vi "Animal Data Top Stack.vi"(2 "State Stack (in)":T1[](array[typedef])) -> (0 "State Stack (out)":T1[](array[typedef]), 1 "State":T1)   [LabVIEW 2016]
uses:
  Animal Data Processor state.ctl
panel:
  # "Top Stack\nVER 1.0 AAM 10th April 2002\n\nThis VI removes the top element of the state stack \nand returns the remaining elements in the stack"
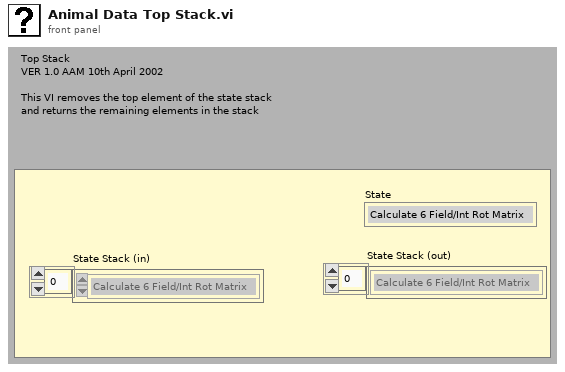
[diagram p1: front panel]
types:
  T1 = typedef "Animal Data Processor state.ctl" = enum16{"Calculate 6 Field/Int Rot Matrix", "Panel Monitoring", "Initialize", "Read 6 Field/Int Calibration File", "Read 6 Field/Int Data File", "Sort 6 Field/Int Channels", "Export Channels", "Stop", "Quit"}
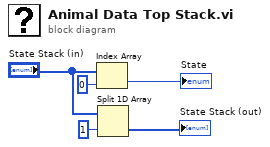
[diagram p0: block diagram]
diagram:
  n1 = Index Array(array="State Stack (in)", index=0) -> (element=→"State":T1)
  n2 = Split 1D Array(array="State Stack (in)", index=1) -> (second subarray=→"State Stack (out)":T1[])  [unwired: 1 out]
